vi "Write Find and Rejoin.vi"(8 "error in":errorcluster, 10 "Find and Rejoin":refnum<notifier>, 11 "Generic Optimization in":refnum<class "Generic Optimization.lvclass">) -> (0 "error out":errorcluster, 3 "Generic Optimization out":refnum<class "Generic Optimization.lvclass">)   [LabVIEW 2018, in "Generic Optimization Actor.lvlib" / "Generic Optimization.lvclass"]
uses:
  Generic Optimization.lvclass
  <vilib>/ActorFramework/Time-Delayed Send Message/Time-Delay Override Options.ctl
  Generic Optimization.lvclass/Generic Optimization.ctl
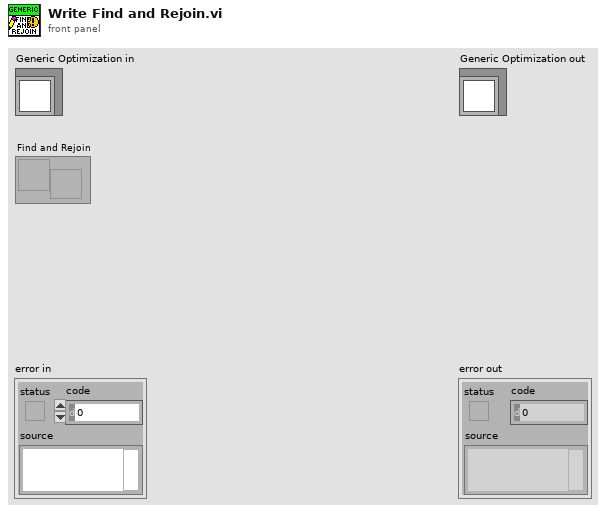
[diagram p1: front panel]
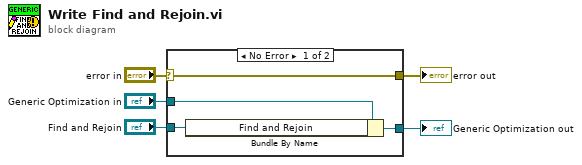
[diagram p0: block diagram]
diagram:
  n1 = case shown="No Error" "error in" {
    selector: "error in" -> [w9 w10]
    tunnel: [w9 w10] -> w4
    tunnel: [w7 w11] -> w2
    tunnel: "Generic Optimization in" -> [w8 w11]
    tunnel: "Find and Rejoin" -> [w6 _]
    frame No Error {
      n2 = Bundle By Name(cluster=w8, "Find and Rejoin"=w6) -> (w7:refnum<class "Generic Optimization.lvclass">)
    }
    frame Error {
    }
  }
  "error out" <- w4
  "Generic Optimization out" <- w2
